vi "1 PPS.vi"() -> (8 "1PPS":bool, 13 "Fractional Seconds":dbl format="%.9f")   [LabVIEW 2023]
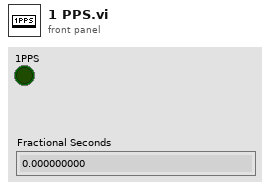
[diagram p1: front panel]
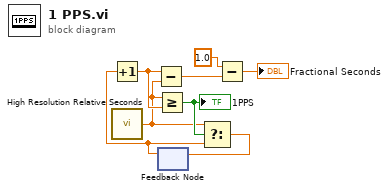
[diagram p0: block diagram]
diagram:
  n1 = call <vilib>:"High Resolution Relative Seconds.vi"() -> ("relative seconds"=w3:dbl)
  n2 = feedback #1() -> (w2:dbl)  [unwired: 1 in]
  n3 = Increment(x=w2) -> (x+1=w4:dbl)
  n4 = Subtract(x=w4, y=w3) -> (x-y=w7:dbl)
  n5 = Greater Or Equal?(x=w3, y=w4) -> (x >= y?=w5:bool)
  "1PPS" <- w5
  n6 = Select(t=w3, s=w5, f=w2) -> (s? t:f=w1:dbl)
  n7 = feedback-in #1(w1) -> ()
  n8 = Subtract(x=1.0, y=w7) -> (x-y=→"Fractional Seconds":dbl)
